vi "Get Configuration Default.vi"(8 "error in (no error)":errorcluster) -> (0 "error out":errorcluster, 3 "Measurement Configuration Default":T1)   [LabVIEW 2020, in "LoadRegulation.lvlib"]
uses:
  LoadRegulation.lvlib
  Measurement Configuration.ctl
  e54118e4-a0f5-41b8-bd23-fc2d3fb72aa9.vi
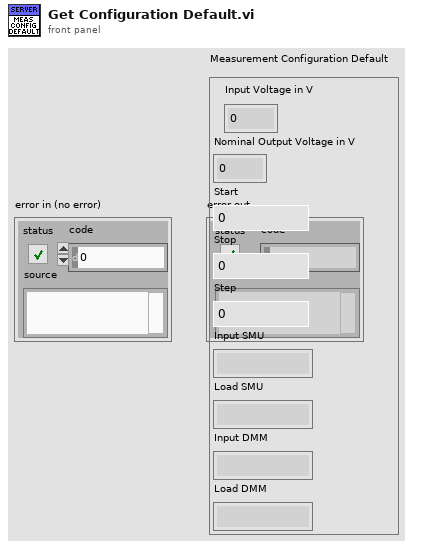
[diagram p1: front panel]
types:
  T1 = typedef "LoadRegulation.lvlib/Measurement Configuration.ctl" = cluster{"Input Voltage in V":dbl, "Nominal Output Voltage in V":dbl, "Start":dbl, "Stop":dbl, "Step":dbl, "Input SMU":string, "Load SMU":string, "Input DMM":string, "Load DMM":string}
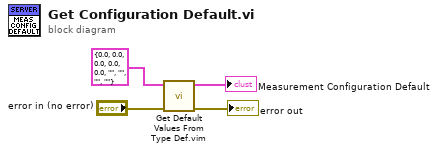
[diagram p0: block diagram]
diagram:
  n1 = call "Get Default Values From Type Def.vim"("error in (no error)"="error in (no error)", "Type Def"=T1 {"Input Voltage in V"=0.0, "Nominal Output Voltage in V"=0.0, "Start"=0.0, "Stop"=0.0, "Step"=0.0, "Input SMU"="", "Load SMU"="", "Input DMM"="", "Load DMM"=""} ("Measurement Configuration")) -> ("error out"=→"error out":errorcluster, "Default Values"=→"Measurement Configuration Default":T1)  [unwired: 8 in]
